vi "MotorInit.vi"(3 "Motor":string="PI1-SHUTTER", 9 "error in (no error)":errorcluster) -> (0 "Motor out":string="PI1-SHUTTER", 1 "Ok?":refnum<k4>, 6 "error out":errorcluster)   [LabVIEW 2009]
uses:
  Controls/MotorCommand.ctl
  Controls/MotorCommandBasic.ctl
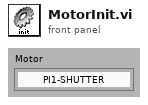
[diagram p1: front panel]
types:
  T1 = typedef "MotorCommandBasic.ctl" = enum16{"SELECT", "MOVE", "PREMOVE", "TURBO", "POS", "NAMED", "INIT", "STOP", "OFF", "SPEED", "QUIT"}
  T2 = typedef "MotorCommand.ctl" = cluster{"Motor":string, "Command":T1, "Movement":i32, "Name":string, "Param":cluster{"VMIN":i32, "VMAX":i32, "ACC":i32}, "Ok?":refnum<k4>, "Go!":refnum<k4>}
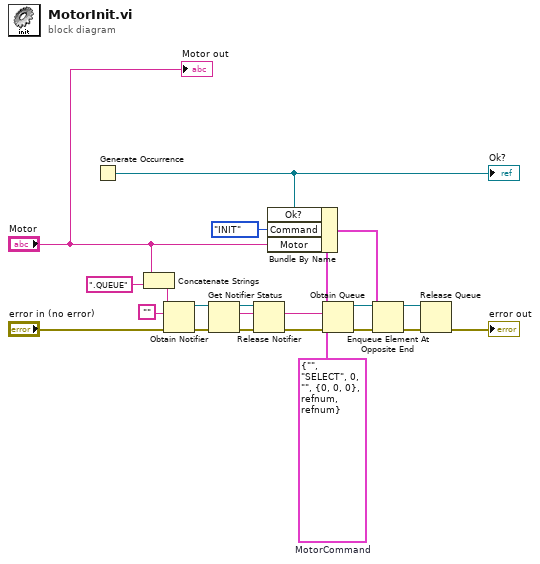
[diagram p0: block diagram]
diagram:
  w18 = T2 {"Motor"="", "Command"=enum."SELECT", "Movement"=0, "Name"="", "Param"={"VMIN"=0, "VMAX"=0, "ACC"=0}, "Ok?"=refnum, "Go!"=refnum}  # MotorCommand
  n1 = Generate Occurrence() -> (w2:refnum<k4>)
  "Ok?" <- w2
  n2 = Concatenate Strings("Motor", ".QUEUE") -> (w9:string)
  n3 = Obtain Notifier(name (unnamed)=w9, notification data type="", error in (no error)="error in (no error)") -> (notifier out=w10:refnum<notifier>, error out=w11:errorcluster)  [unwired: 1 in, 1 out]
  n4 = Get Notifier Status(notifier=w10, error in (no error)=w11) -> (notifier out=w13:refnum<notifier>, current notification=w6:string, error out=w14:errorcluster)  [unwired: 2 out]
  n5 = Release Notifier(notifier=w13, error in (no error)=w14) -> (error out=w7:errorcluster)  [unwired: 3 out]
  n6 = Bundle By Name(cluster=w18, "Ok?"=w2, "Command"=MotorCommandBasic."INIT", "Motor"="Motor") -> (w17:T2)
  n7 = Obtain Queue(name (unnamed)=w6, element data type=w18, error in (no error)=w7) -> (queue out=w20:refnum<queue>, error out=w19:errorcluster)  [unwired: 2 in, 1 out]
  n8 = Enqueue Element At Opposite End(queue=w20, element=w17, error in (no error)=w19) -> (queue out=w15:refnum<queue>, error out=w16:errorcluster)  [unwired: 2 out]
  n9 = Release Queue(queue=w15, error in (no error)=w16) -> (error out=→"error out":errorcluster)  [unwired: 3 out]
  "Motor out" <- "Motor"
